vi "m100Output.vi"(8 "error in (no error)":errorcluster, 10 "Input":string[][](array[string]), 11 "report in":refnum<class "NI_report.lvclass">) -> (0 "error out":errorcluster, 3 "report out":refnum<class "NI_report.lvclass">)   [LabVIEW 2012]
uses:
  <vilib>/Utility/NIReport.llb/NI_report.lvclass
  <vilib>/Utility/NIReport.llb/Append Text Table to Report (wrap).vi
  <vilib>/Utility/NIReport.llb/Excel/NI_Excel.lvclass
  <vilib>/addons/_office/NI_ReportGenerationToolkit.lvlib
panel:
  in  "Header":string
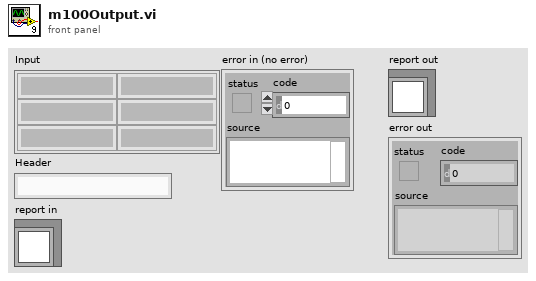
[diagram p1: front panel]
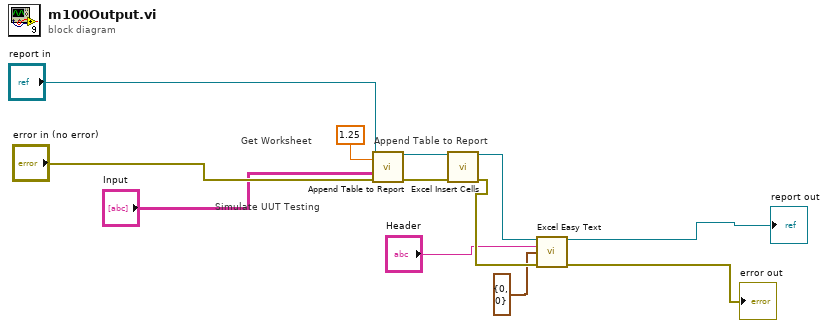
[diagram p0: block diagram]
diagram:
  # "Simulate UUT Testing"
  # "Append Table to Report"
  # "Get Worksheet"
  n1 = call-poly <vilib>:"Append Table to Report.vi"("report in"="report in", "column width (1)"=1.25, "text data"="Input", "error in (no error)"="error in (no error)") -> ("report out"=w11:refnum<class "NI_report.lvclass">, "error out"=w10:errorcluster)  [unwired: 8 in, 2 out]
  n2 = call <vilib>:"Excel Insert Cells.vi"("report in"=w11, "error in (no error)"=w10) -> ("report out"=w9:refnum<class "NI_report.lvclass">, "error out"=w8:errorcluster)  [unwired: 12 in]
  n3 = call <vilib>:"Excel Easy Text.vi"("report in"=w9, "text"="Header", "start (-1, -1)"=cluster{"row":i32, "column":i32} {"row"=0, "column"=0} ("end (-1, -1)"), "error in (no error)"=w8) -> ("report out"=→"report out":refnum<class "NI_report.lvclass">, "error out"=→"error out":errorcluster)  [unwired: 7 in, 3 out]
